vi "Decode Pixel.vi"(9 "B":u8(slide) scale=0.0..255.0, 10 "G":u8(slide) scale=0.0..255.0, 11 "R":u8(slide) scale=0.0..255.0) -> (3 "Bits":bool[](array[boolean]))   [LabVIEW 2020]
panel:
  out "Avg":i32(slide) scale=0.0..255.0
  out "Source Color":u32(colorbox)
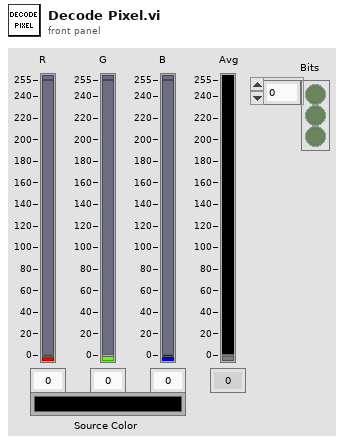
[diagram p1: front panel]
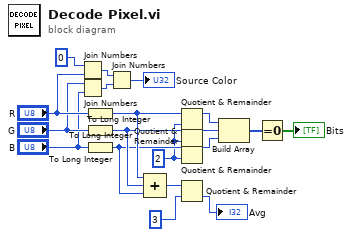
[diagram p0: block diagram]
diagram:
  w1 = 2 ("y")
  n1 = Join Numbers(hi=u8 0, lo="R") -> ((hi.lo)=w19:u16)
  n2 = Join Numbers(hi="G", lo="B") -> ((hi.lo)=w18:u16)
  n3 = To Long Integer(number="R") -> (32bit integer=w9:i32)
  n4 = To Long Integer(number="G") -> (32bit integer=w8:i32)
  n5 = To Long Integer(number="B") -> (32bit integer=w7:i32)
  n6 = Join Numbers(hi=w19, lo=w18) -> ((hi.lo)=→"Source Color":u32)
  n7 = Compound Arithmetic op=ADD(w9, w8, w7) -> (w12:i32)
  n8 = Quotient & Remainder(x=w9, y=w1) -> (x-y*floor(x/y)=w4:i32)  [unwired: 1 out]
  n9 = Quotient & Remainder(x=w8, y=w1) -> (x-y*floor(x/y)=w6:i32)  [unwired: 1 out]
  n10 = Quotient & Remainder(x=w7, y=w1) -> (x-y*floor(x/y)=w5:i32)  [unwired: 1 out]
  n11 = Quotient & Remainder(x=w12, y=3) -> (floor(x/y)=→"Avg":i32)  [unwired: 1 out]
  n12 = Build Array(w4, w6, w5) -> (w3:i32[])
  n13 = Equal To 0?(x=w3) -> (x = 0?=→"Bits":bool[])
